vi "calc waveforms.vi"() -> (1 "do waveforms":T5[](array[typedef]))   [LabVIEW 2015]
uses:
  type def/NI card channels.ctl
  type def/do waveform.ctl
  type def/basic params.ctl
  type def/advanced params.ctl
  type def/PXI control.ctl
  <instrlib>/niScope/Controls/niScope trigger source digital.ctl
  global variables/params.vi
panel:
  out "line trigger 3":i16[](graph)
  out "line trigger 2":i16[](graph)
  out "synchonize":i16[](graph)
  out "line trigger":i16[](graph)
  out "x galvo waveform":dbl[](graph)
  in  "y galvo 0":i32=32800
  in  "x galvo 0":i32=31800
  in  "PXI channel":T1={"Vertical Range (V)"=1.0, "Min Sample Rate"=2208791.906743315, "# of Channels"=1, "Min Record Length"=560, "Number Of Records"=10000, "Trigger Position(%)"=0.0, "act Record Length"=1000, "trigger source"="VAL_EXTERNAL", "PMT2 # of Channels"=1} {"PMT2 # of Channels" min=1 max=8 step=1; "act Record Length" min=0 max=100 format="%#.3g"; "Trigger Position(%)" min=0.0 max=1000000.0 step=1.0 format="%#.3p"; "Number Of Records" min=0 max=10000 step=1 format="%#.3g"; "Min Record Length" min=1 max=8 step=1; "# of Channels" min=1 max=8 step=1; "Min Sample Rate" min=0.0 max=100000000.0 format="%#.3p"; "Vertical Range (V)" min=0.0 max=10.0 format="%#.3g"}
  in  "advanced params":T3={"x flyback time(%)"=40.0, "signal offset"=0, "frame time(s)"=0.0, "fetch # per frame"=1, "galvo sampling rate"=500000} {"galvo sampling rate" min=10000 max=200000 step=1; "fetch # per frame" min=1 max=100 step=1 format="%#.3g"; "frame time(s)" min=0.0 max=100.0 step=0.1 format="%#.3g"; "signal offset" max=10000 format="%#.3g"; "x flyback time(%)" min=0.0 max=50.0 format="%#.3g"}
  in  "basic params":T4={"X pixel #"=200, "X pixel size(um)"=1.0, "Y pixel #"=200, "Y pixel size(um)"=10.0, "line rate(Hz)"=1.0, "stage scan?"=FALSE} {"line rate(Hz)" min=1.0 max=2000.0 format="%#.3g"; "X pixel size(um)" min=0.0 max=10.0 format="%#.3g"; "X pixel #" min=2 max=20480 step=2 format="%#.3g"; "Y pixel size(um)" min=0.0 max=10.0 format="%#.3g"; "Y pixel #" min=2 max=204800 step=2 format="%#.3g"}
  in  "galvo y flyback pixel #":u32
  in  "galvo x flyback pixel #":u32
  in  "galvo x pixel #":u32
  out "y galvo waveform":dbl[](graph)
  in  "NI card channels":T6=[{"signal"="x galvo", "DAQmx Physical Channel"="Dev1/ao0", "max"=10.0, "min"=-10.0, "DAQmx Terminal"="", "start trigger"="", "ClockSource"="", "Scaling Factor"=1.0, "Notes"=""}, {"signal"="y galvo", "DAQmx Physical Channel"="Dev1/ao1", "max"=10.0, "min"=-10.0, "DAQmx Terminal"="", "start trigger"="", "ClockSource"="", "Scaling Factor"=1.0, "Notes"=""}]
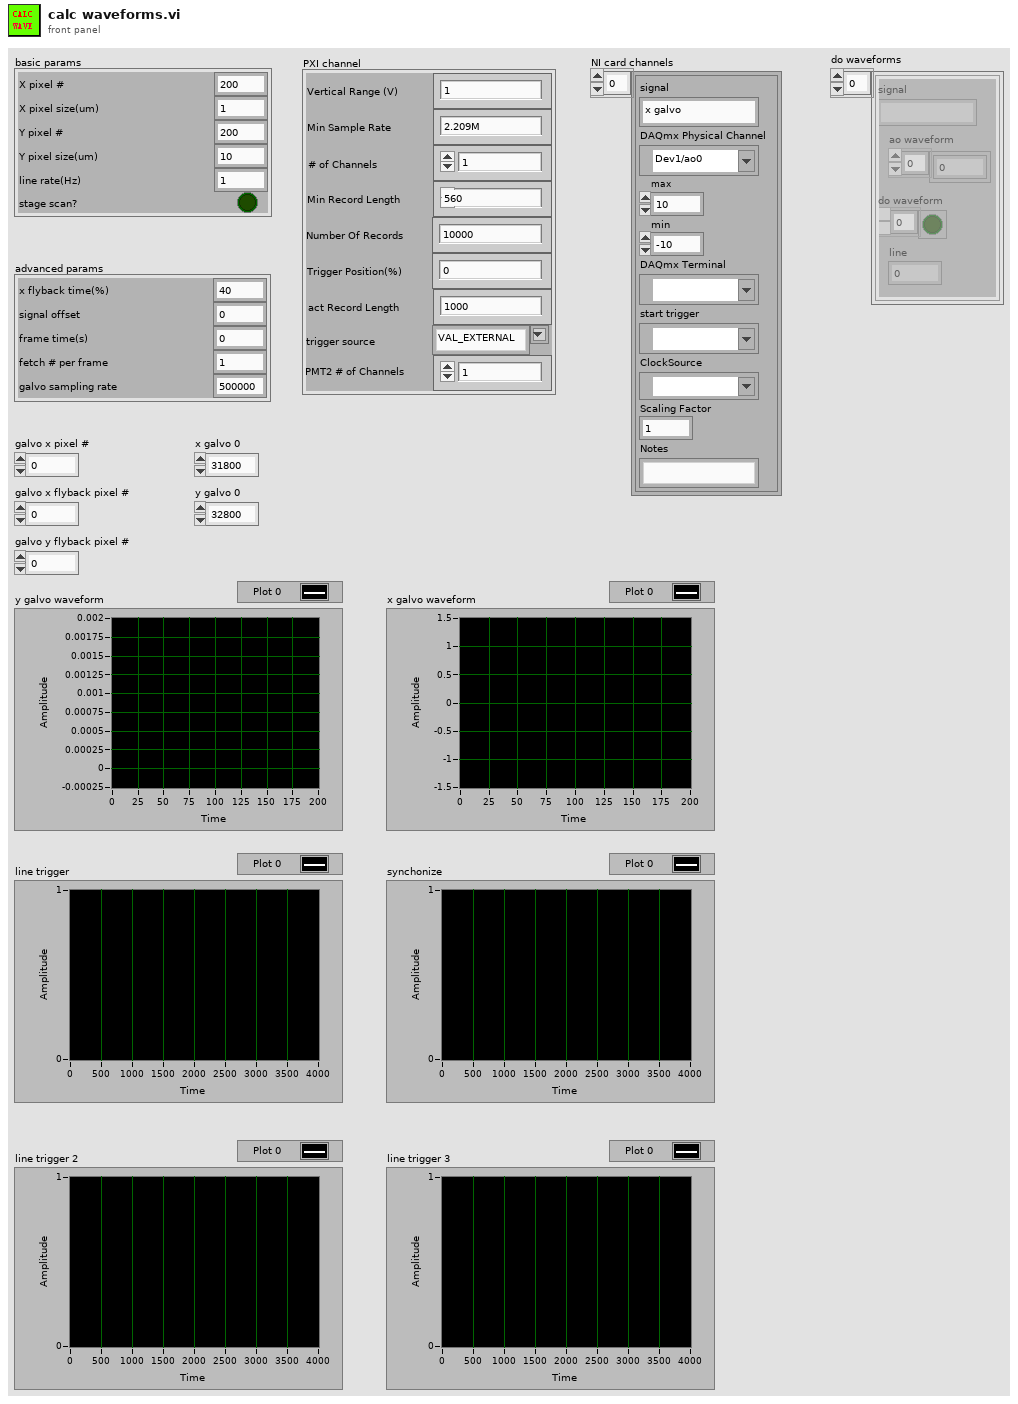
[diagram p1: front panel]
types:
  T1 = typedef "PXI control.ctl" = cluster{"Vertical Range (V)":dbl, "Min Sample Rate":dbl, "# of Channels":u8, "Min Record Length":i32, "Number Of Records":i32, "Trigger Position(%)":dbl, "act Record Length":i32, "trigger source":T2, "PMT2 # of Channels":u8}
  T2 = typedef "niScope trigger source digital.ctl" = string
  T3 = typedef "advanced params.ctl" = cluster{"x flyback time(%)":dbl, "signal offset":u16, "frame time(s)":dbl, "fetch # per frame":u16, "galvo sampling rate":u32}
  T4 = typedef "basic params.ctl" = cluster{"X pixel #":u32, "X pixel size(um)":dbl, "Y pixel #":u32, "Y pixel size(um)":dbl, "line rate(Hz)":dbl, "stage scan?":bool}
  T5 = typedef "do waveform.ctl" = cluster{"signal":string, "ao waveform":dbl[], "do waveform":bool[], "line":u8}
  T6 = typedef "NI card channels.ctl" = cluster{"signal":string, "DAQmx Physical Channel":tag, "max":dbl, "min":dbl, "DAQmx Terminal":tag, "start trigger":tag, "ClockSource":tag, "Scaling Factor":dbl, "Notes":string}[]
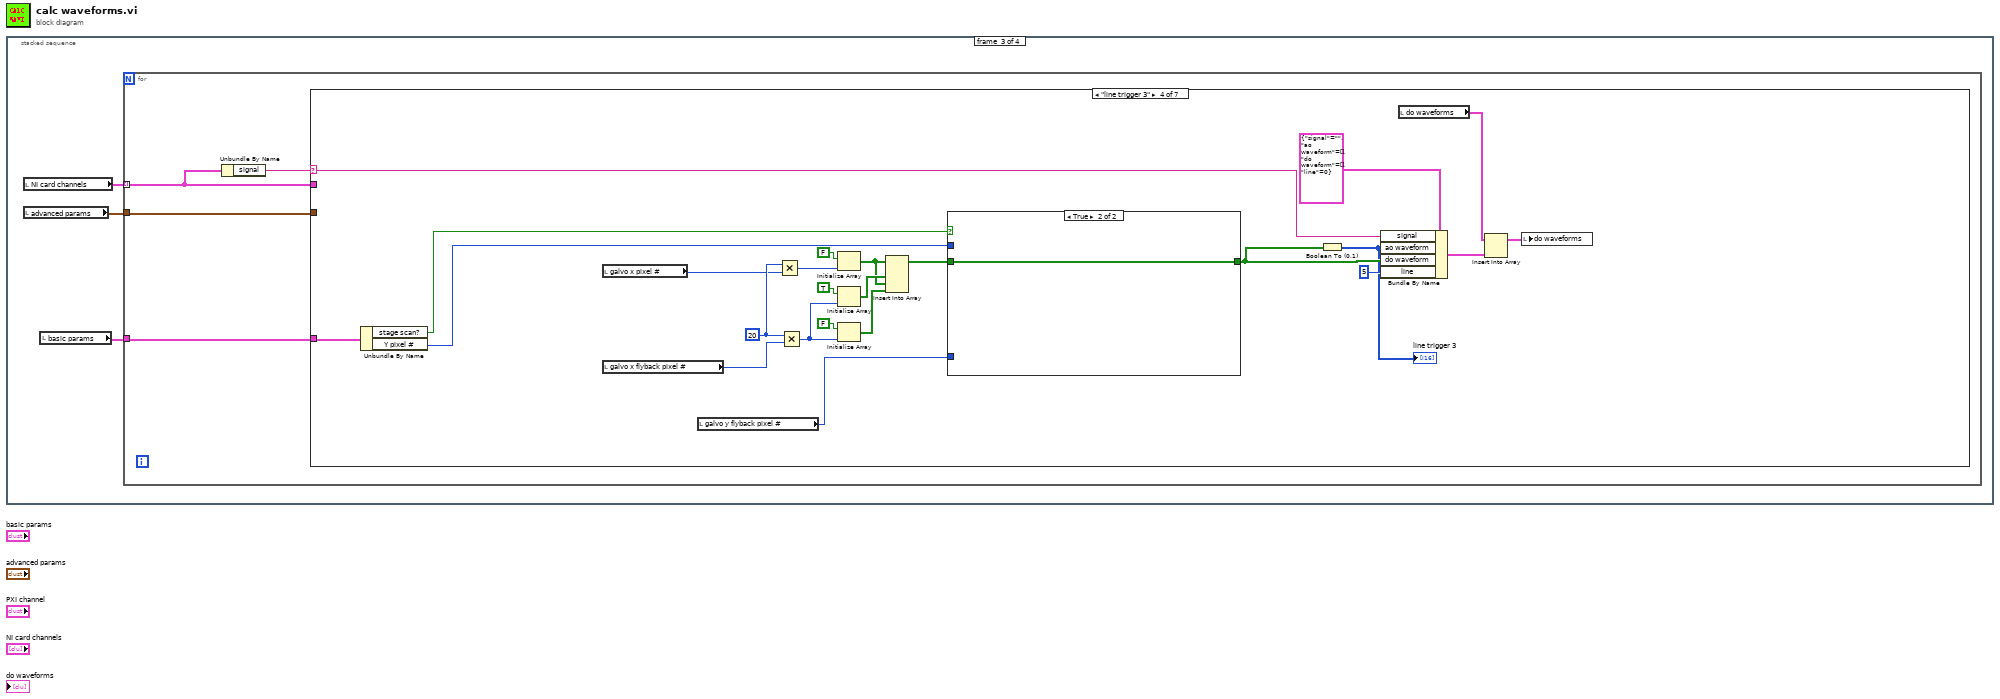
[diagram p0: block diagram]
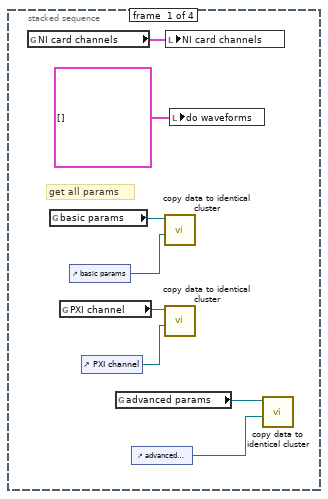
[diagram p2: hidden frame]
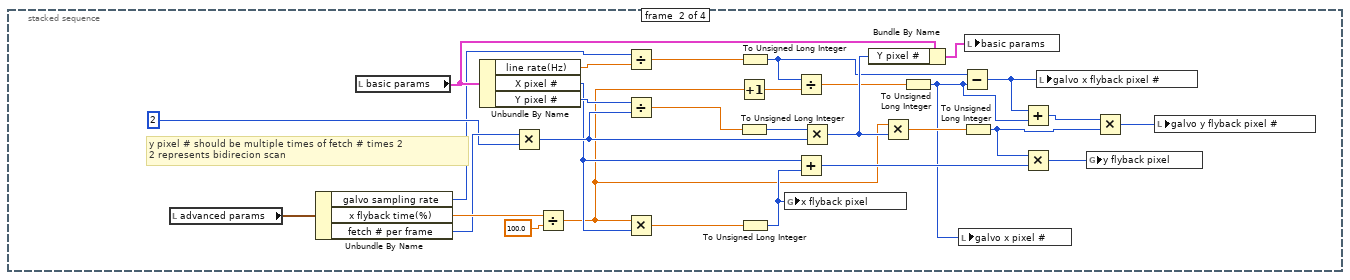
[diagram p3: hidden frame]
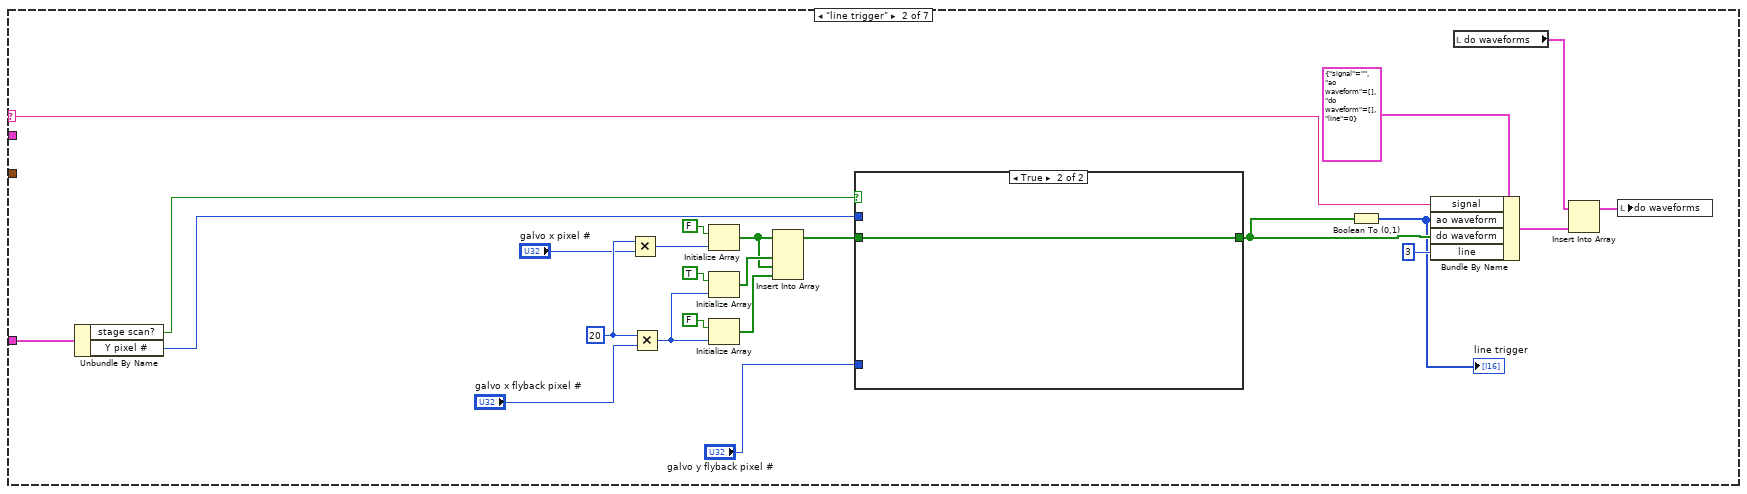
[diagram p5: hidden frame]
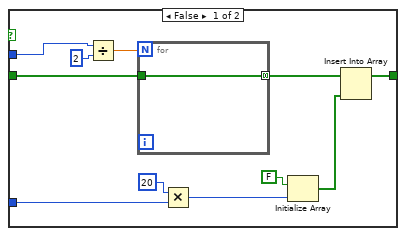
[diagram p6: hidden frame]
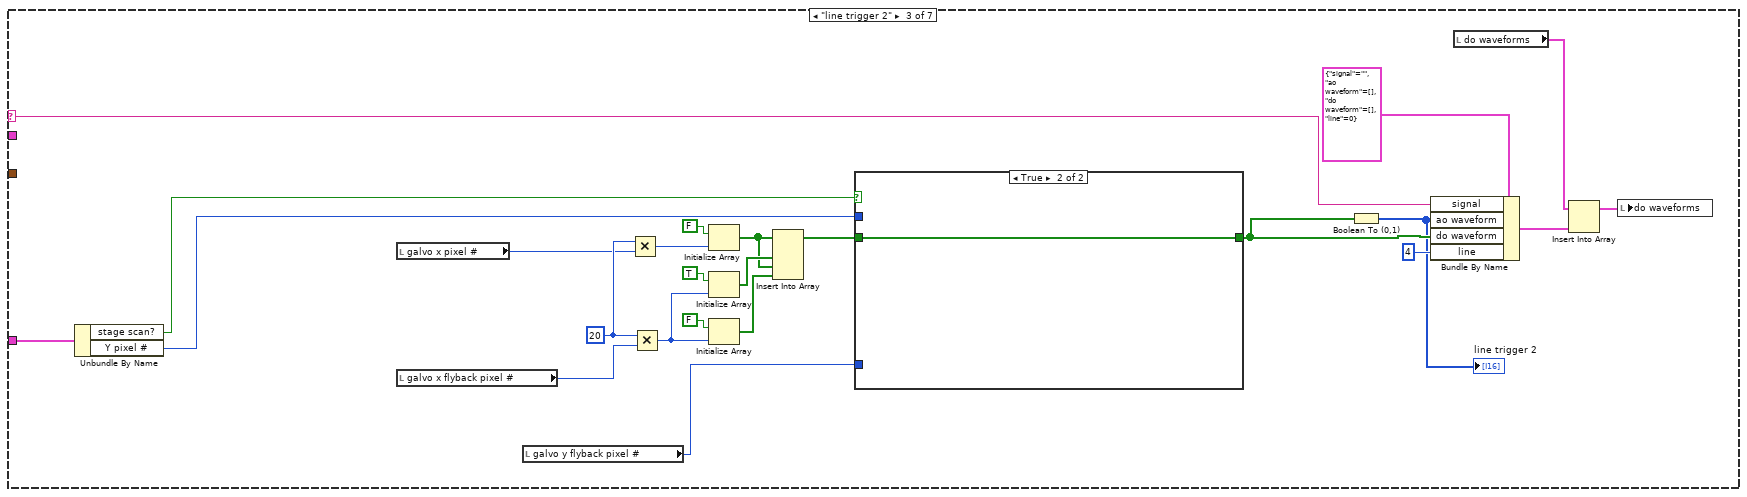
[diagram p7: hidden frame]
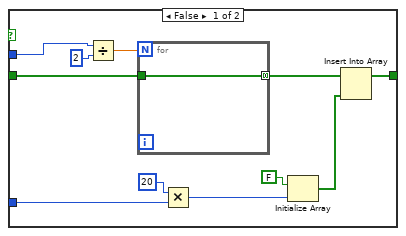
[diagram p8: hidden frame]
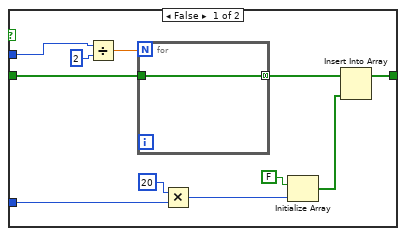
[diagram p9: hidden frame]
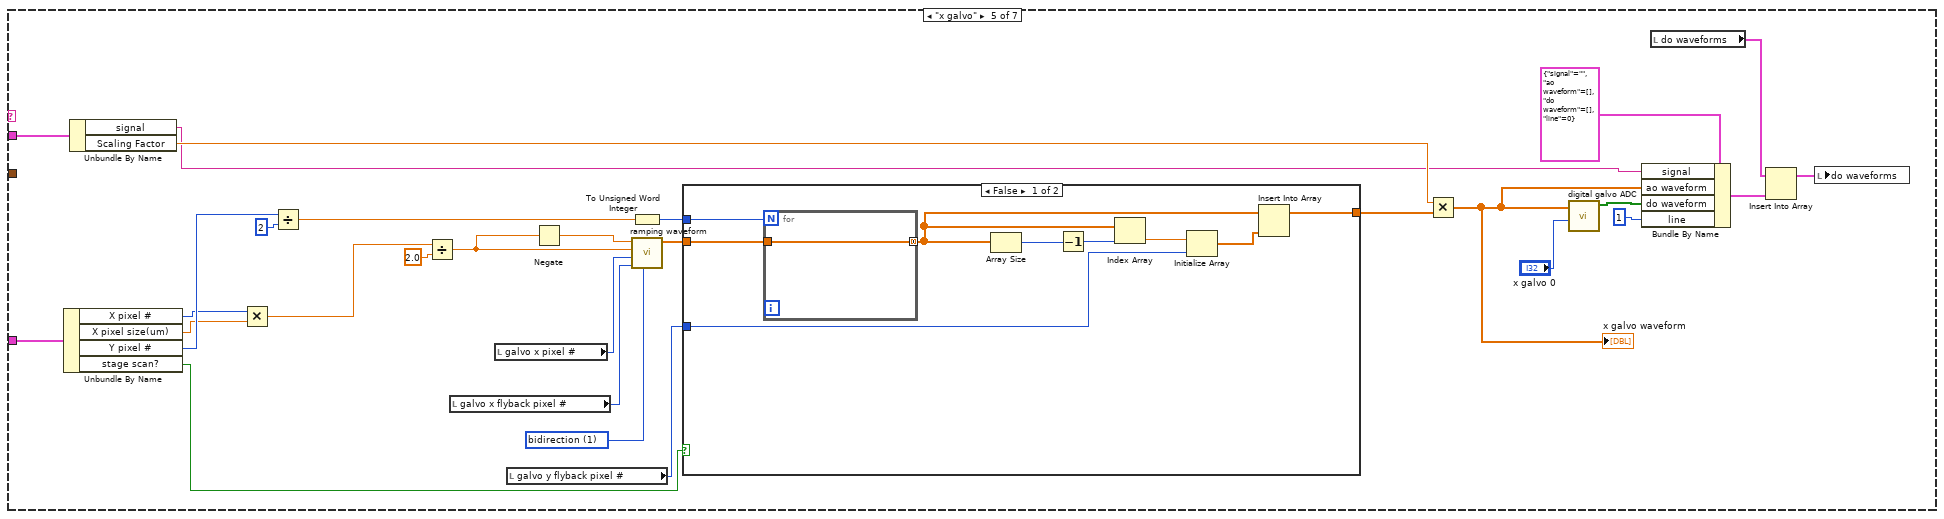
[diagram p10: hidden frame]
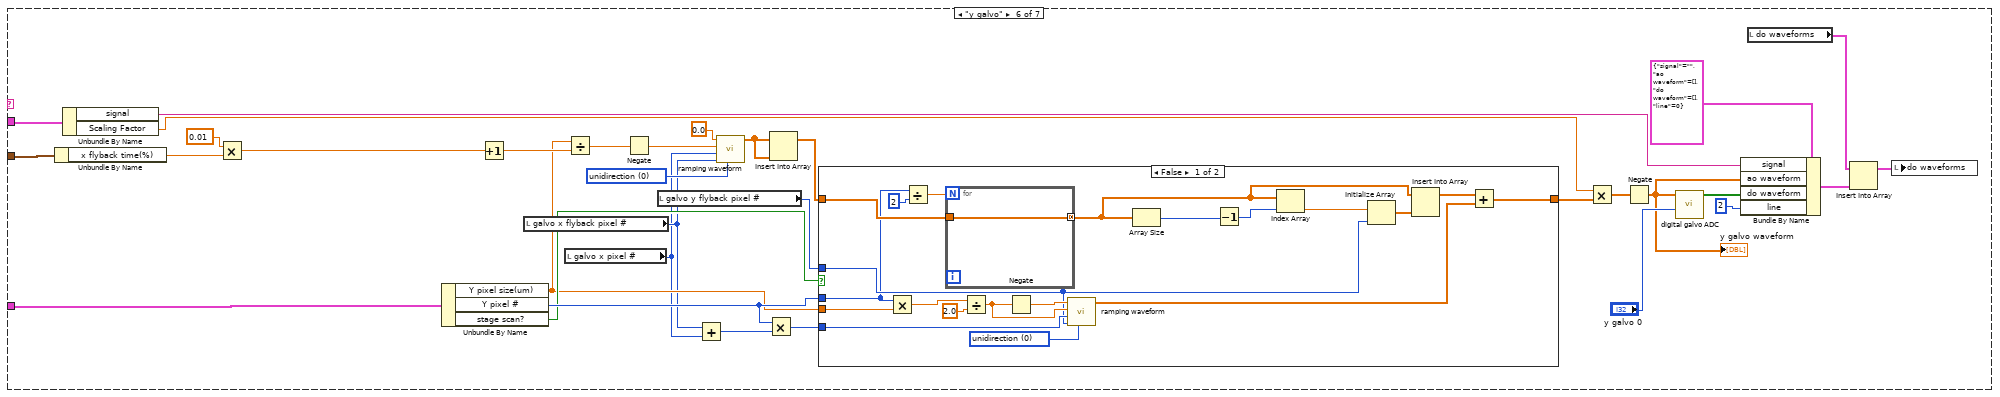
[diagram p12: hidden frame]
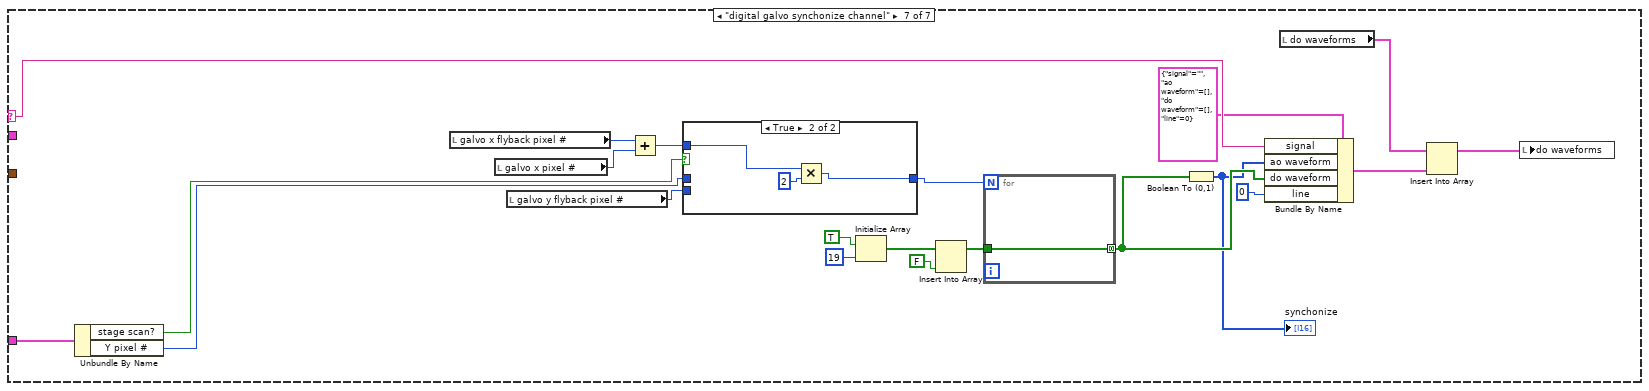
[diagram p14: hidden frame]
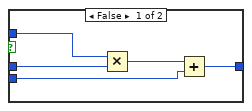
[diagram p15: hidden frame]
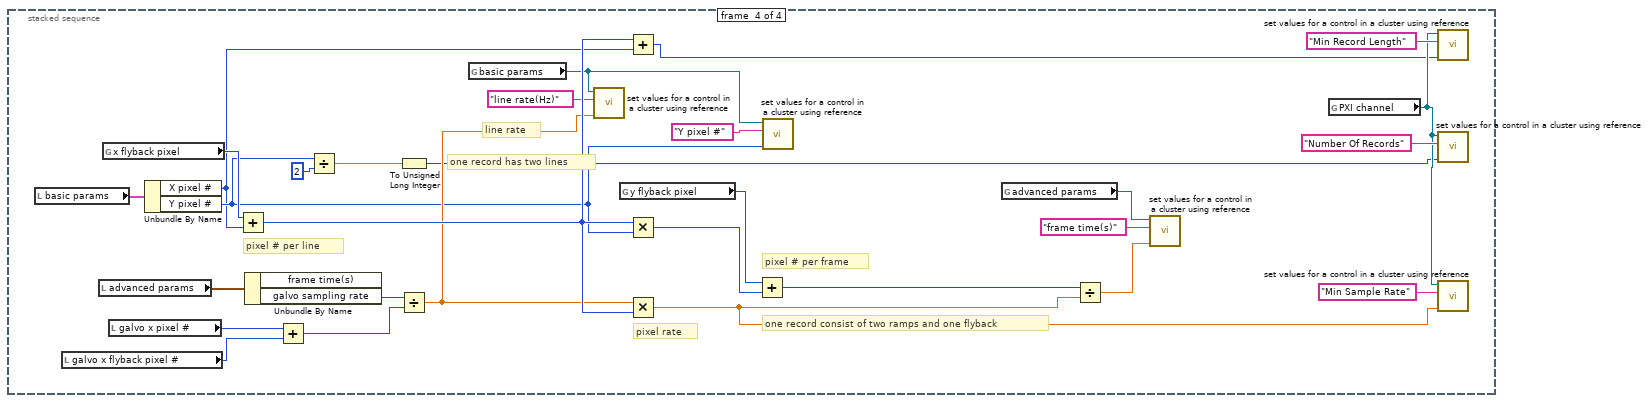
[diagram p16: hidden frame]
diagram:
  n1 = stacked-sequence {
    frame #0 {
      # "get all params"
      n2 = global read "params.vi" "NI card channels"() -> (w6:T6)
      n3 = global read "params.vi" "basic params"() -> (w7:refnum<vi>)
      n4 = global read "params.vi" "PXI channel"() -> (w5:refnum<vi>)
      n5 = control-ref of="basic params"() -> (w3:refnum<vi>)
      n6 = control-ref of="PXI channel"() -> (w1:refnum<vi>)
      n7 = global read "params.vi" "advanced params"() -> (w8:refnum<vi>)
      n8 = control-ref of="advanced params"() -> (w2:refnum<vi>)
      n9 = call "copy data to identical cluster.vi"("Guest Clust Refnum"=w3, "Host Clust Refnum"=w7) -> ()  [unwired: 10 in]
      n10 = call "copy data to identical cluster.vi"("Guest Clust Refnum"=w1, "Host Clust Refnum"=w5) -> ()  [unwired: 10 in]
      n11 = local write "NI card channels"(w6) -> ()
      n12 = local write "do waveforms"(T5[] [] ("dev0 do waveform")) -> ()
      n13 = call "copy data to identical cluster.vi"("Guest Clust Refnum"=w2, "Host Clust Refnum"=w8) -> ()  [unwired: 10 in]
    }
    frame #1 {
      # "y pixel # should be multiple times of fetch # times 2\n2 represents bidirecion scan"
      n14 = local read "advanced params"() -> (w38:T3)
      n15 = Unbundle By Name(w38) -> ("galvo sampling rate"=w20:u32, "x flyback time(%)"=w37:dbl, "fetch # per frame"=w28:u16)
      n16 = local read "basic params"() -> (w30:T4)
      n17 = Unbundle By Name(w30) -> ("line rate(Hz)"=w19:dbl, "X pixel #"=w23:u32, "Y pixel #"=w34:u32)
      n18 = Multiply(x=w28, y=u32 2) -> (x*y=w27:u32)
      n19 = Divide(x=w37, y=100.0) -> (x/y=w17:dbl)
      n20 = Divide(x=w20, y=w19) -> (x/y=w18:dbl)
      n21 = Divide(x=w34, y=w27) -> (x/y=w33:dbl)
      n22 = Multiply(x=w17, y=w23) -> (x*y=w36:dbl)
      n23 = Increment(x=w17) -> (x+1=w16:dbl)
      n24 = To Unsigned Long Integer(number=w33) -> (unsigned 32bit integer=w32:u32)
      n25 = To Unsigned Long Integer(number=w18) -> (unsigned 32bit integer=w14:u32)
      n26 = To Unsigned Long Integer(number=w36) -> (unsigned 32bit integer=w24:u32)
      n27 = global write "params.vi" "x flyback pixel"(w24) -> ()
      n28 = Divide(x=w14, y=w16) -> (x/y=w15:dbl)
      n29 = Add(x=w23, y=w24) -> (x+y=w22:u32)
      n30 = Multiply(x=w32, y=w27) -> (x*y=w25:u32)
      n31 = Bundle By Name(cluster=w30, "Y pixel #"=w25) -> (w29:T4)
      n32 = Multiply(x=w17, y=w25) -> (x*y=w31:dbl)
      n33 = To Unsigned Long Integer(number=w15) -> (unsigned 32bit integer=w12:u32)
      n34 = local write "galvo x pixel #"(w12) -> ()
      n35 = Subtract(x=w14, y=w12) -> (x-y=w13:u32)
      n36 = To Unsigned Long Integer(number=w31) -> (unsigned 32bit integer=w10:u32)
      n37 = local write "basic params"(w29) -> ()
      n38 = Add(x=w13, y=w12) -> (x+y=w11:u32)
      n39 = Multiply(x=w10, y=w22) -> (x*y=w21:u32)
      n40 = local write "galvo x flyback pixel #"(w13) -> ()
      n41 = global write "params.vi" "y flyback pixel"(w21) -> ()
      n42 = Multiply(x=w11, y=w10) -> (x*y=w9:u32)
      n43 = local write "galvo y flyback pixel #"(w9) -> ()
    }
    frame #2 {
      n44 = local read "NI card channels"() -> (w41:T6)
      n45 = local read "advanced params"() -> (w39:T3)
      n46 = local read "basic params"() -> (w40:T4)
      n47 = for {
        tunnel: w41 -> [w42] mode=indexing
        tunnel: w40 -> [w44]
        tunnel: w39 -> [w43]
        n48 = Unbundle By Name(w42) -> ("signal"=w45:string)
        n49 = case shown="\"line trigger 3\"" w45 {
          selector: w45 -> [_ w68 w105 w142 _ _ w271]
          tunnel: w44 -> [_ w69 w106 w143 w174 w223 w272]
          tunnel: w43 -> [_ _ _ _ _ w213 _]
          tunnel: w42 -> [_ _ _ _ w162 w203 _]
          frame "False", Default {
          }
          frame "line trigger" {
            w51 = u32 20 ("x")
            n50 = Unbundle By Name(w69) -> ("stage scan?"=w62:bool, "Y pixel #"=w61:u32)
            n51 = Multiply(x=w51, y="galvo x pixel #") -> (x*y=w52:u32)
            n52 = Multiply(x=w51, y="galvo x flyback pixel #") -> (x*y=w50:u32)
            n53 = Initialize Array(FALSE, w52) -> (w56:bool[])
            n54 = Initialize Array(TRUE, w50) -> (w58:bool[])
            n55 = Initialize Array(FALSE, w50) -> (w54:bool[])
            n56 = Insert Into Array(array=w56, new element #1=w58, new element #2=w56, new element #3=w54) -> (w57:bool[])  [unwired: 1 in]
            n57 = case shown="True" w62 {
              tunnel: w61 -> [w71 _]
              tunnel: "galvo y flyback pixel #" -> [w75 _]
              tunnel: w57 -> [w80 w82]
              tunnel: [w76 w82] -> w53
              frame False {
                n58 = Divide(x=w71, y=u32 2) -> (x/y=w70:dbl)
                n59 = for {
                  N: w70 -> [_]
                  tunnel: w80 -> [w81]
                  tunnel: [w81] -> w78 mode=concatenating
                }
                n60 = Multiply(x=u32 20, y=w75) -> (x*y=w74:u32)
                n61 = Initialize Array(FALSE, w74) -> (w77:bool[])
                n62 = Insert Into Array(array=w78, new element=w77) -> (w76:bool[])  [unwired: 1 in]
              }
              frame True {
              }
            }
            n63 = Boolean To (0,1)(Boolean=w53) -> (0, 1=w46:i16[])
            "line trigger" <- w46
            n64 = Bundle By Name(cluster=T5 {"signal"="", "ao waveform"=[], "do waveform"=[], "line"=0} ("dev0 do waveform"), "signal"=w68, "ao waveform"=w46, "do waveform"=w53, "line"=u8 3) -> (w64:T5)
            n65 = local read "do waveforms"() -> (w65:T5[])
            n66 = Insert Into Array(array=w65, new element=w64) -> (w63:T5[])  [unwired: 1 in]
            n67 = local write "do waveforms"(w63) -> ()
          }
          frame "line trigger 2" {
            w88 = u32 20 ("x")
            n68 = Unbundle By Name(w106) -> ("stage scan?"=w99:bool, "Y pixel #"=w98:u32)
            n69 = local read "galvo x pixel #"() -> (w85:u32)
            n70 = local read "galvo x flyback pixel #"() -> (w84:u32)
            n71 = local read "galvo y flyback pixel #"() -> (w83:u32)
            n72 = Multiply(x=w88, y=w85) -> (x*y=w89:u32)
            n73 = Multiply(x=w88, y=w84) -> (x*y=w87:u32)
            n74 = Initialize Array(FALSE, w89) -> (w93:bool[])
            n75 = Initialize Array(TRUE, w87) -> (w95:bool[])
            n76 = Initialize Array(FALSE, w87) -> (w91:bool[])
            n77 = Insert Into Array(array=w93, new element #1=w95, new element #2=w93, new element #3=w91) -> (w94:bool[])  [unwired: 1 in]
            n78 = case shown="True" w99 {
              tunnel: w98 -> [w108 _]
              tunnel: w83 -> [w112 _]
              tunnel: w94 -> [w117 w119]
              tunnel: [w113 w119] -> w90
              frame False {
                n79 = Divide(x=w108, y=u32 2) -> (x/y=w107:dbl)
                n80 = for {
                  N: w107 -> [_]
                  tunnel: w117 -> [w118]
                  tunnel: [w118] -> w115 mode=concatenating
                }
                n81 = Multiply(x=u32 20, y=w112) -> (x*y=w111:u32)
                n82 = Initialize Array(FALSE, w111) -> (w114:bool[])
                n83 = Insert Into Array(array=w115, new element=w114) -> (w113:bool[])  [unwired: 1 in]
              }
              frame True {
              }
            }
            n84 = Boolean To (0,1)(Boolean=w90) -> (0, 1=w86:i16[])
            "line trigger 2" <- w86
            n85 = Bundle By Name(cluster=T5 {"signal"="", "ao waveform"=[], "do waveform"=[], "line"=0} ("dev0 do waveform"), "signal"=w105, "ao waveform"=w86, "do waveform"=w90, "line"=u8 4) -> (w101:T5)
            n86 = local read "do waveforms"() -> (w102:T5[])
            n87 = Insert Into Array(array=w102, new element=w101) -> (w100:T5[])  [unwired: 1 in]
            n88 = local write "do waveforms"(w100) -> ()
          }
          frame "line trigger 3" {
            w125 = u32 20 ("x")
            n89 = Unbundle By Name(w143) -> ("stage scan?"=w136:bool, "Y pixel #"=w135:u32)
            n90 = local read "galvo x pixel #"() -> (w122:u32)
            n91 = local read "galvo x flyback pixel #"() -> (w121:u32)
            n92 = local read "galvo y flyback pixel #"() -> (w120:u32)
            n93 = Multiply(x=w125, y=w122) -> (x*y=w126:u32)
            n94 = Multiply(x=w125, y=w121) -> (x*y=w124:u32)
            n95 = Initialize Array(FALSE, w126) -> (w130:bool[])
            n96 = Initialize Array(TRUE, w124) -> (w132:bool[])
            n97 = Initialize Array(FALSE, w124) -> (w128:bool[])
            n98 = Insert Into Array(array=w130, new element #1=w132, new element #2=w130, new element #3=w128) -> (w131:bool[])  [unwired: 1 in]
            n99 = case shown="True" w136 {
              tunnel: w135 -> [w145 _]
              tunnel: w120 -> [w149 _]
              tunnel: w131 -> [w154 w156]
              tunnel: [w150 w156] -> w127
              frame False {
                n100 = Divide(x=w145, y=u32 2) -> (x/y=w144:dbl)
                n101 = for {
                  N: w144 -> [_]
                  tunnel: w154 -> [w155]
                  tunnel: [w155] -> w152 mode=concatenating
                }
                n102 = Multiply(x=u32 20, y=w149) -> (x*y=w148:u32)
                n103 = Initialize Array(FALSE, w148) -> (w151:bool[])
                n104 = Insert Into Array(array=w152, new element=w151) -> (w150:bool[])  [unwired: 1 in]
              }
              frame True {
              }
            }
            n105 = Boolean To (0,1)(Boolean=w127) -> (0, 1=w123:i16[])
            "line trigger 3" <- w123
            n106 = Bundle By Name(cluster=T5 {"signal"="", "ao waveform"=[], "do waveform"=[], "line"=0} ("dev0 do waveform"), "signal"=w142, "ao waveform"=w123, "do waveform"=w127, "line"=u8 5) -> (w138:T5)
            n107 = local read "do waveforms"() -> (w139:T5[])
            n108 = Insert Into Array(array=w139, new element=w138) -> (w137:T5[])  [unwired: 1 in]
            n109 = local write "do waveforms"(w137) -> ()
          }
          frame "x galvo" {
            w178 = u16 1 items=["unidirection", "bidirection"] ("mode")
            n110 = Unbundle By Name(w174) -> ("X pixel #"=w175:u32, "X pixel size(um)"=w177:dbl, "Y pixel #"=w181:u32, "stage scan?"=w173:bool)
            n111 = Unbundle By Name(w162) -> ("signal"=w159:string, "Scaling Factor"=w161:dbl)
            n112 = Multiply(x=w175, y=w177) -> (x*y=w185:dbl)
            n113 = Divide(x=w181, y=u32 2) -> (x/y=w180:dbl)
            n114 = Divide(x=w185, y=2.0) -> (x/y=w182:dbl)
            n115 = local read "galvo x flyback pixel #"() -> (w165:u32)
            n116 = local read "galvo x pixel #"() -> (w163:u32)
            n117 = local read "galvo y flyback pixel #"() -> (w164:u32)
            n118 = Negate(x=w182) -> (-x=w183:dbl)
            n119 = To Unsigned Word Integer(number=w180) -> (unsigned 16bit integer=w172:u16)
            n120 = call "ramping waveform.vi"("mode"=w178, "points in t2"=w165, "points in t1"=w163, "p2"=w182, "p1"=w183) -> ("array"=w176:dbl[])  [unwired: 6 in]
            n121 = case shown="False" w173 {
              tunnel: w176 -> [w194 w196]
              tunnel: [w192 w196] -> w160
              tunnel: w172 -> [w190 _]
              tunnel: w164 -> [w186 _]
              frame False {
                n122 = for {
                  N: w190 -> [_]
                  tunnel: w194 -> [w195]
                  tunnel: [w195] -> w189 mode=concatenating
                }
                n123 = Array Size(array=w189) -> (size(s)=w188:i32)
                n124 = Decrement(x=w188) -> (x-1=w187:i32)
                n125 = Index Array(array=w189, index=w187) -> (element=w193:dbl)
                n126 = Initialize Array(w193, w186) -> (w191:dbl[])
                n127 = Insert Into Array(array=w189, new element=w191) -> (w192:dbl[])  [unwired: 1 in]
              }
              frame True {
              }
            }
            n128 = Multiply(x=w161, y=w160) -> (x*y=w157:dbl[])
            "x galvo waveform" <- w157
            n129 = call "digital galvo ADC.vi"("zero point"="x galvo 0", "Analog waveform"=w157) -> ("Digital waveform"=w170:bool[])  [unwired: 9 in]
            n130 = Bundle By Name(cluster=T5 {"signal"="", "ao waveform"=[], "do waveform"=[], "line"=0} ("dev0 do waveform"), "signal"=w159, "ao waveform"=w157, "do waveform"=w170, "line"=u8 1) -> (w167:T5)
            n131 = local read "do waveforms"() -> (w168:T5[])
            n132 = Insert Into Array(array=w168, new element=w167) -> (w166:T5[])  [unwired: 1 in]
            n133 = local write "do waveforms"(w166) -> ()
          }
          frame "y galvo" {
            w229 = u16 0 items=["unidirection", "bidirection"] ("mode")
            n134 = Unbundle By Name(w213) -> ("x flyback time(%)"=w212:dbl)
            n135 = Unbundle By Name(w203) -> ("signal"=w199:string, "Scaling Factor"=w202:dbl)
            n136 = Multiply(x=0.01, y=w212) -> (x*y=w210:dbl)
            n137 = Unbundle By Name(w223) -> ("Y pixel size(um)"=w208:dbl, "Y pixel #"=w222:u32, "stage scan?"=w214:bool)
            n138 = Increment(x=w210) -> (x+1=w209:dbl)
            n139 = local read "galvo x flyback pixel #"() -> (w206:u32)
            n140 = local read "galvo x pixel #"() -> (w205:u32)
            n141 = Divide(x=w208, y=w209) -> (x/y=w207:dbl)
            n142 = Negate(x=w207) -> (-x=w215:dbl)
            n143 = local read "galvo y flyback pixel #"() -> (w204:u32)
            n144 = Add(x=w206, y=w205) -> (x+y=w225:u32)
            n145 = call "ramping waveform.vi"("mode"=w229, "points in t2"=w206, "points in t1"=w205, "p2"=w215, "p1"=0.0) -> ("array"=w227:dbl[])  [unwired: 6 in]
            n146 = Multiply(x=w222, y=w225) -> (x*y=w224:u32)
            n147 = Insert Into Array(array=w227, new element=w227) -> (w226:dbl[])  [unwired: 1 in]
            n148 = case shown="False" w214 {
              tunnel: w226 -> [w249 w251]
              tunnel: [w235 w251] -> w201
              tunnel: w208 -> [w246 _]
              tunnel: w224 -> [w241 _]
              tunnel: w204 -> [w239 _]
              tunnel: w222 -> [w233 _]
              frame False {
                w234 = u16 0 items=["unidirection", "bidirection"] ("mode")
                n149 = Multiply(x=w233, y=w246) -> (x*y=w245:dbl)
                n150 = Divide(x=w233, y=u32 2) -> (x/y=w247:dbl)
                n151 = for {
                  N: w247 -> [_]
                  tunnel: w249 -> [w250]
                  tunnel: [w250] -> w232 mode=concatenating
                }
                n152 = Divide(x=w245, y=2.0) -> (x/y=w242:dbl)
                n153 = Negate(x=w242) -> (-x=w243:dbl)
                n154 = call "ramping waveform.vi"("mode"=w234, "points in t2"=w239, "points in t1"=w241, "p2"=w242, "p1"=w243) -> ("array"=w236:dbl[])  [unwired: 6 in]
                n155 = Array Size(array=w232) -> (size(s)=w231:i32)
                n156 = Decrement(x=w231) -> (x-1=w230:i32)
                n157 = Index Array(array=w232, index=w230) -> (element=w240:dbl)
                n158 = Initialize Array(w240, w239) -> (w238:dbl[])
                n159 = Insert Into Array(array=w232, new element=w238) -> (w237:dbl[])  [unwired: 1 in]
                n160 = Add(x=w237, y=w236) -> (x+y=w235:dbl[])
              }
              frame True {
              }
            }
            n161 = Multiply(x=w202, y=w201) -> (x*y=w200:dbl[])
            n162 = Negate(x=w200) -> (-x=w197:dbl[])
            "y galvo waveform" <- w197
            n163 = call "digital galvo ADC.vi"("zero point"="y galvo 0", "Analog waveform"=w197) -> ("Digital waveform"=w220:bool[])  [unwired: 9 in]
            n164 = Bundle By Name(cluster=T5 {"signal"="", "ao waveform"=[], "do waveform"=[], "line"=0} ("dev0 do waveform"), "signal"=w199, "ao waveform"=w197, "do waveform"=w220, "line"=u8 2) -> (w217:T5)
            n165 = local read "do waveforms"() -> (w218:T5[])
            n166 = Insert Into Array(array=w218, new element=w217) -> (w216:T5[])  [unwired: 1 in]
            n167 = local write "do waveforms"(w216) -> ()
          }
          frame "digital galvo synchonize channel" {
            n168 = Unbundle By Name(w272) -> ("stage scan?"=w256:bool, "Y pixel #"=w255:u32)
            n169 = local read "galvo x flyback pixel #"() -> (w258:u32)
            n170 = local read "galvo x pixel #"() -> (w257:u32)
            n171 = local read "galvo y flyback pixel #"() -> (w254:u32)
            n172 = Add(x=w258, y=w257) -> (x+y=w265:u32)
            n173 = case shown="True" w256 {
              tunnel: w265 -> [w277 w280]
              tunnel: w255 -> [w276 _]
              tunnel: w254 -> [w274 _]
              tunnel: [w273 w278] -> w253
              frame False {
                n174 = Multiply(x=w277, y=w276) -> (x*y=w275:u32)
                n175 = Add(x=w275, y=w274) -> (x+y=w273:u32)
              }
              frame True {
                n176 = Multiply(x=w280, y=u16 2) -> (x*y=w278:u32)
              }
            }
            n177 = Initialize Array(TRUE, 19 ("dimension size")) -> (w262:bool[])
            n178 = Insert Into Array(array=w262, new element=FALSE) -> (w264:bool[])  [unwired: 1 in]
            n179 = for {
              N: w253 -> [_]
              tunnel: w264 -> [w281]
              tunnel: [w281] -> w259 mode=concatenating
            }
            n180 = Boolean To (0,1)(Boolean=w259) -> (0, 1=w252:i16[])
            "synchonize" <- w252
            n181 = Bundle By Name(cluster=T5 {"signal"="", "ao waveform"=[], "do waveform"=[], "line"=0} ("dev0 do waveform"), "signal"=w271, "ao waveform"=w252, "do waveform"=w259, "line"=u8 0) -> (w267:T5)
            n182 = local read "do waveforms"() -> (w268:T5[])
            n183 = Insert Into Array(array=w268, new element=w267) -> (w266:T5[])  [unwired: 1 in]
            n184 = local write "do waveforms"(w266) -> ()
          }
        }
      }
    }
    frame #3 {
      # "one record has two lines"
      # "one record consist of two ramps and one flyback"
      # "line rate"
      # "pixel rate"
      # "pixel # per frame"
      # "pixel # per line"
      n185 = local read "basic params"() -> (w305:T4)
      n186 = local read "galvo x flyback pixel #"() -> (w294:u32)
      n187 = local read "advanced params"() -> (w303:T3)
      n188 = global read "params.vi" "x flyback pixel"() -> (w301:u16)
      n189 = local read "galvo x pixel #"() -> (w293:u32)
      n190 = Unbundle By Name(w305) -> ("X pixel #"=w282:u32, "Y pixel #"=w287:u32)
      n191 = Add(x=w301, y=w282) -> (x+y=w297:u32)
      n192 = Unbundle By Name(w303) -> ("galvo sampling rate"=w292:u32)  [unwired: 1 out]
      n193 = Add(x=w293, y=w294) -> (x+y=w291:u32)
      n194 = Divide(x=w287, y=u32 2) -> (x/y=w285:dbl)
      n195 = To Unsigned Long Integer(number=w285) -> (unsigned 32bit integer=w283:u32)
      n196 = Divide(x=w292, y=w291) -> (x/y=w289:dbl)
      n197 = global read "params.vi" "basic params"() -> (w288:refnum<vi>)
      n198 = call "set values for a control in a cluster using reference.vi"("value"=w289, "name"="line rate(Hz)", "Clust Refnum"=w288) -> ()  [unwired: 9 in]
      n199 = global read "params.vi" "y flyback pixel"() -> (w299:u16)
      n200 = Add(x=w297, y=w282) -> (x+y=w296:u32)
      n201 = Multiply(x=w297, y=w287) -> (x*y=w300:u32)
      n202 = Multiply(x=w289, y=w297) -> (x*y=w295:dbl)
      n203 = Add(x=w299, y=w300) -> (x+y=w284:u32)
      n204 = call "set values for a control in a cluster using reference.vi"("value"=w287, "name"="Y pixel #", "Clust Refnum"=w288) -> ()  [unwired: 9 in]
      n205 = global read "params.vi" "advanced params"() -> (w302:refnum<vi>)
      n206 = Divide(x=w284, y=w295) -> (x/y=w298:dbl)
      n207 = call "set values for a control in a cluster using reference.vi"("value"=w298, "name"="frame time(s)", "Clust Refnum"=w302) -> ()  [unwired: 9 in]
      n208 = global read "params.vi" "PXI channel"() -> (w307:refnum<vi>)
      n209 = call "set values for a control in a cluster using reference.vi"("value"=w296, "name"="Min Record Length", "Clust Refnum"=w307) -> ()  [unwired: 9 in]
      n210 = call "set values for a control in a cluster using reference.vi"("value"=w283, "name"="Number Of Records", "Clust Refnum"=w307) -> ()  [unwired: 9 in]
      n211 = call "set values for a control in a cluster using reference.vi"("value"=w295, "name"="Min Sample Rate", "Clust Refnum"=w307) -> ()  [unwired: 9 in]
    }
  }
